vi "Create ErrorMsg.vi"(8 "error in (no error)":errorcluster, 10 "Error Cluster":errorcluster, 11 "Message Name":string) -> (0 "error out":errorcluster, 3 "ErrorMsg out":refnum<class "ErrorMsg.lvclass">)   [LabVIEW 2017, in "LapDog.Messaging.v3.lvlib" / "ErrorMsg.lvclass"]
doc: "Creates an ErrorMsg object with the given name. If no name is given the message name is the same as the class name.\n\nThis method executes regardless of the error in state."
uses:
  ErrorMsg.lvclass
  C:/git/LapDog.Messaging/src/LapDog.Messaging/Message/Message.lvclass
  Message/Message.lvclass
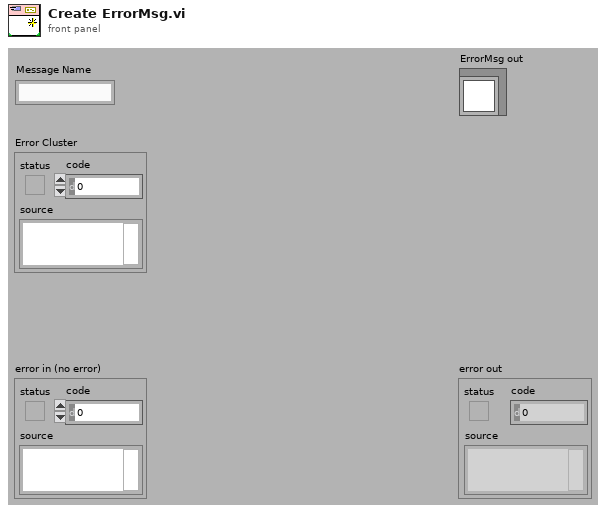
[diagram p1: front panel]
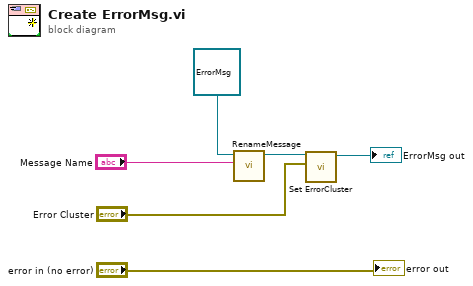
[diagram p0: block diagram]
diagram:
  n1 = call "RenameMessage.vi"("Message Name"="Message Name", "Message in"=refnum<class "ErrorMsg.lvclass"> refnum ("ErrorMsg in")) -> ("Message out"=w3:refnum<class "ErrorMsg.lvclass">)  [unwired: 8 in, 1 out]
  n2 = call-dynamic "Set ErrorCluster.vi"("ErrorCluster"="Error Cluster", "ErrorMsg in"=w3) -> ("ErrorMsg out"=→"ErrorMsg out":refnum<class "ErrorMsg.lvclass">)  [unwired: 8 in, 1 out]
  "error out" <- "error in (no error)"
